vi "Creating_Backup_SQL.vi"(8 "error in":errorcluster, 10 "User level":i32, 11 "database in":T1) -> (0 "error out":errorcluster, 2 "User Level":i32, 3 "Database out":T1)   [LabVIEW 2017]
doc: "This vi we used to create SQL backup and delete that backup from SQL. This backup is moved to to CSV file.."
uses:
  <vilib>/addons/database/Connection.llb/Conn ObjectReference.ctl
  <vilib>/Utility/config.llb/Read Key (Path).vi
  <vilib>/Utility/config.llb/Read Key (Double).vi
  <vilib>/Utility/config.llb/Read Key (Boolean).vi
  <vilib>/Utility/file.llb/Write Delimited Spreadsheet (string).vi
  <vilib>/addons/database/NI_Database_API.lvlib
  <vilib>/Utility/config.llb/NI_LVConfig.lvlib
panel:
  out "Get Backup\nTreshold Time":timestamp caption="Get Backup Treshold Time"
  out "Backup Treshold Days":u32
  out "From Date":string
  in  "TO DATE":timestamp format="%<%d/%m/%Y>T"
  in  "FROM DATE":timestamp format="%<%d/%m/%Y>T"
  out "x*y":dbl
  out "x-y 3":dbl
  out "Backup Treshold Time":timestamp
  out "x-y":dbl
  out "Current Time":timestamp
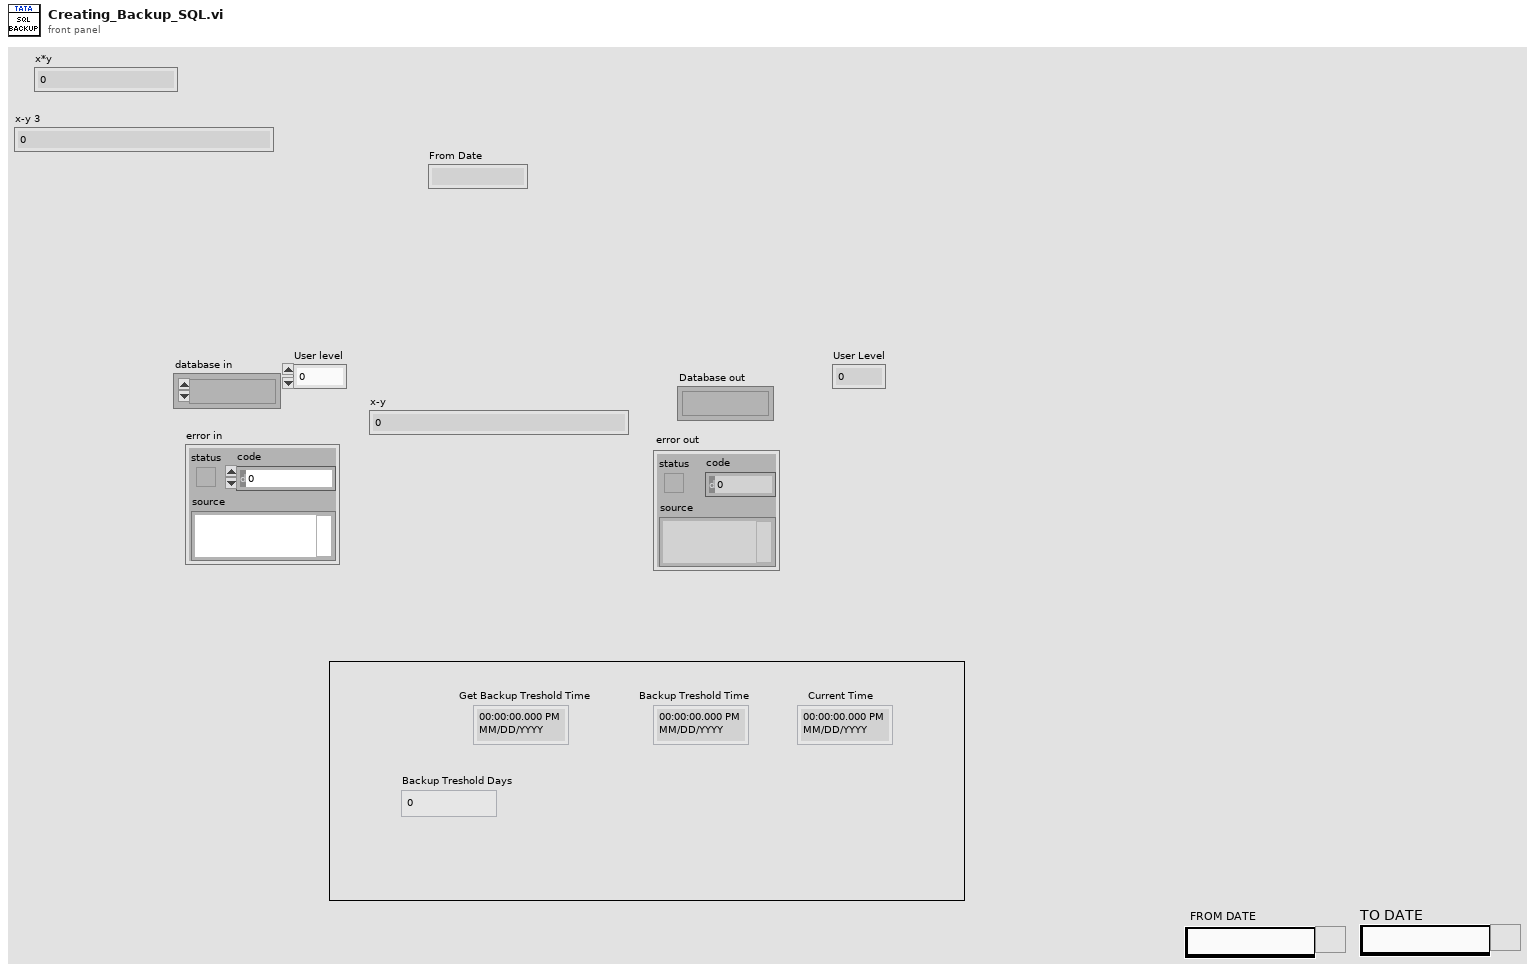
[diagram p1: front panel]
types:
  T1 = typedef "NI_Database_API.lvlib/Conn ObjectReference.ctl" = refnum<k1>
  T2 = enum32{"invalid app kind", "Development System", "Run Time System", "Student Edition", "Embedded LabVIEW", "Evaluation", "Custom"}
  T3 = typedef "NI_LVConfig.lvlib/Config Data RefNum.ctl" = refnum<k1>
  T4 = typedef "LVDateTimeRec.ctl" = cluster{"fractional second":dbl, "second":i32, "minute":i32, "hour":i32, "day of month":i32, "month":i32, "year":i32, "day of week":i32, "day of year":i32, "DST":i32}
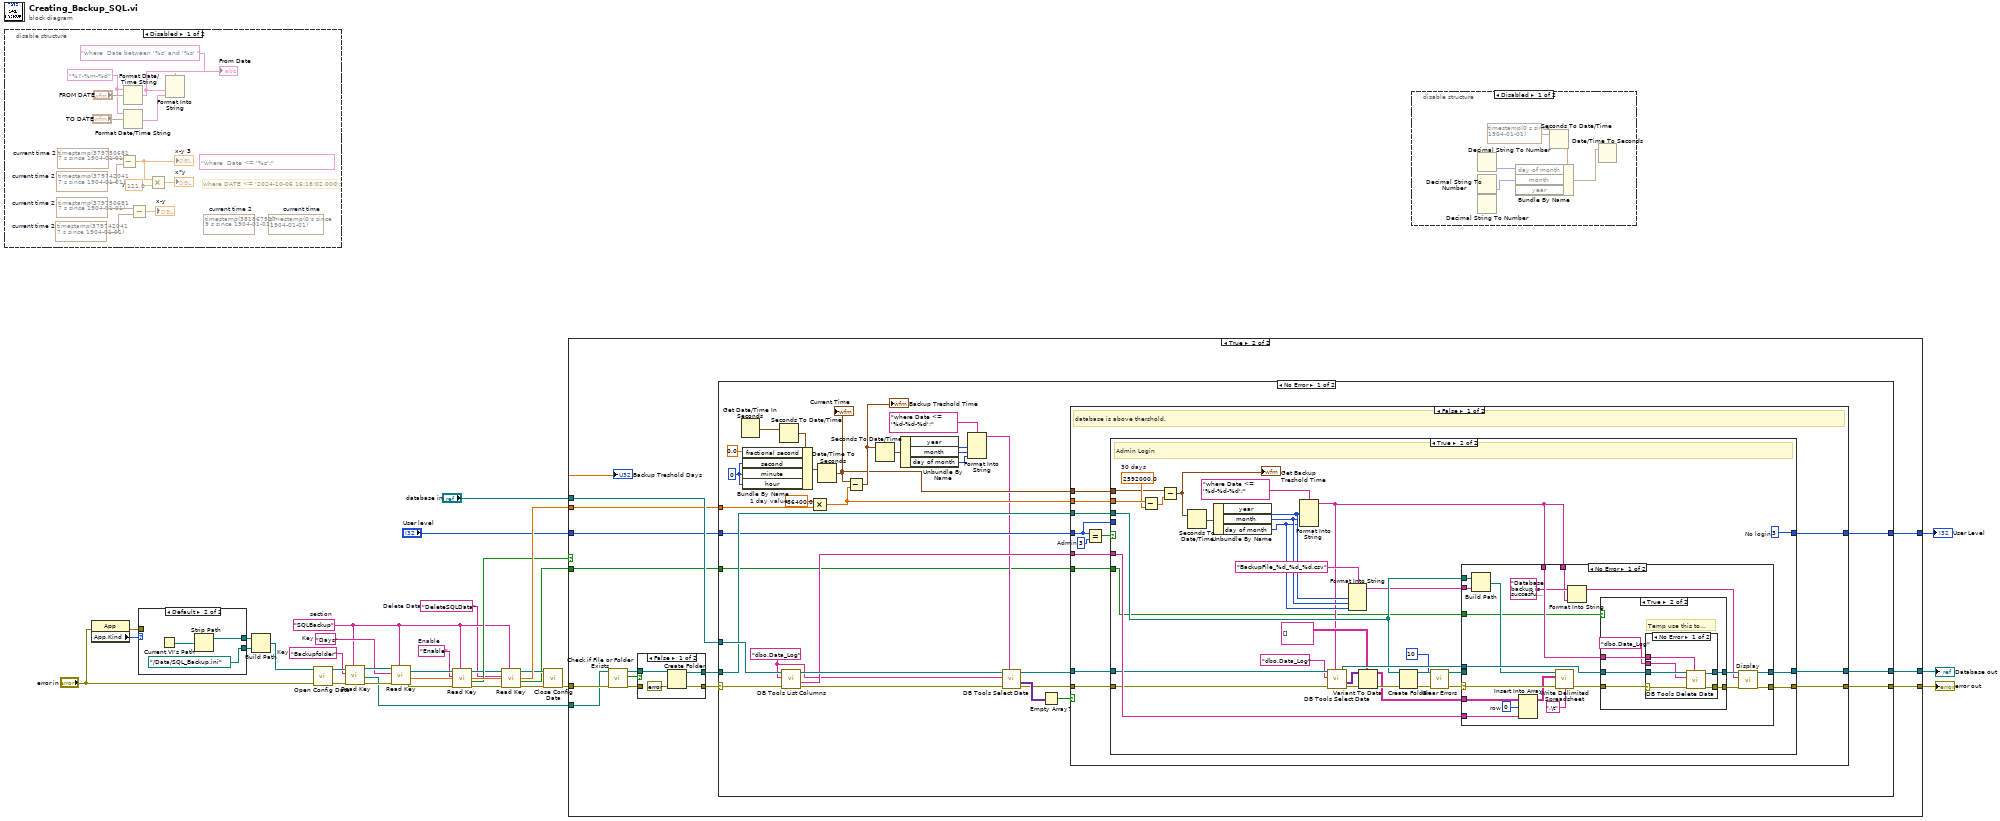
[diagram p0: block diagram]
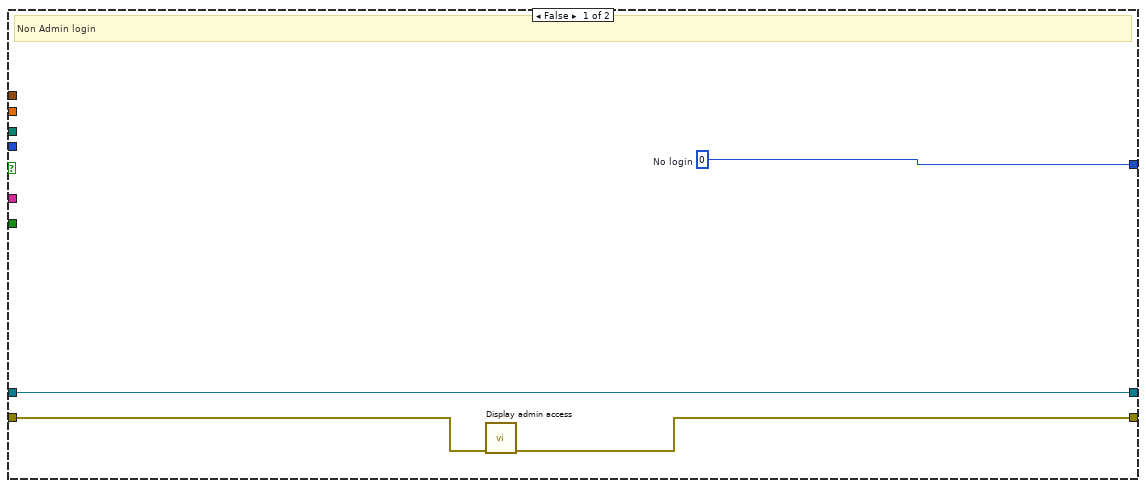
[diagram p4: hidden frame]
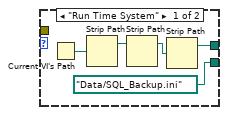
[diagram p12: hidden frame]
diagram:
  w2 = "DeleteSQLData"  # Delete Data
  w9 = "Enable"  # Enable
  w20 = "Days"  # Key
  w21 = "Backupfolder"  # Key
  w3 = "SQLBackup"  # section
  n1 = disable-structure shown="Disabled" {
    frame Disabled {
      w32 = "%Y-%m-%d"
      w39 = 121.0  # y
      w41 = timestamp(3797420417.197 s since 1904-01-01)  # current time 2
      w42 = timestamp(3797506817.197 s since 1904-01-01)  # current time 2
      (unwired) "where  Date <= '%s';" ("format string")
      (unwired) timestamp(3818675179.6780734 s since 1904-01-01)  # current time 2
      w44 = timestamp(3797420417.197 s since 1904-01-01)  # current time 2
      w45 = timestamp(3797506817.197 s since 1904-01-01)  # current time 2
      (unwired) timestamp(0 s since 1904-01-01)  # current time
      # "where DATE <= '2024-10-06 16:18:02.000';"
      n2 = Subtract(x=w42, y=w41) -> (x-y=w40:dbl)
      "x-y 3" <- w40
      n3 = Format Date/Time String(time format string (%c)=w32, seconds (now)="FROM DATE") -> (date/time string=w37:string)  [unwired: 1 in]
      "From Date" <- w37
      n4 = Format Date/Time String(time format string (%c)=w32, seconds (now)="TO DATE") -> (date/time string=w36:string)  [unwired: 1 in]
      n5 = Subtract(x=w45, y=w44) -> (x-y=→"x-y":dbl)
      n6 = Multiply(x=w40, y=w39) -> (x*y=→"x*y":dbl)
      n7 = Format Into String(format string="where  Date between '%s' and '%s' ", w37, w36) -> ()  [unwired: 2 in, 2 out]
    }
    frame Enabled {
    }
  }
  n8 = property class="App"(error in="error in") -> (error out=w28:errorcluster, "App.Kind"=w29:T2)  [unwired: 1 in, 1 out]
  n9 = case shown="Default" w29 {
    tunnel: [w47 w52] -> w27
    tunnel: w28 -> [_ _]
    tunnel: [path "Data/SQL_Backup.ini" ("path") path "../Data/SQL_Backup.ini" ("path")] -> w26
    frame "Run Time System" {
      n10 = Current VI's Path() -> (path=w50:path)
      n11 = Strip Path(path=w50) -> (stripped path=w49:path)  [unwired: 1 out]
      n12 = Strip Path(path=w49) -> (stripped path=w48:path)  [unwired: 1 out]
      n13 = Strip Path(path=w48) -> (stripped path=w47:path)  [unwired: 1 out]
    }
    frame Default {
      n14 = Current VI's Path() -> (path=w53:path)
      n15 = Strip Path(path=w53) -> (stripped path=w52:path)  [unwired: 1 out]
    }
  }
  n16 = Build Path(base path=w27, name or relative path=w26) -> (appended path=w17:path)
  n17 = call <vilib>:"Open Config Data.vi"("error in (no error)"="error in", "configuration file path"=w17) -> ("error out"=w25:errorcluster, "refnum"=w24:T3)  [unwired: 7 in, 1 out]
  n18 = call-poly <vilib>:"Read Key.vi"("section"=w3, "error in (no error)"=w25, "key"=w21, "refnum"=w24) -> ("error out"=w22:errorcluster, "value"=w16:path, "refnum out"=w23:T3)  [unwired: 4 in, 1 out]
  n19 = call-poly <vilib>:"Read Key.vi"("section"=w3, "error in (no error)"=w22, "key"=w20, "refnum"=w23) -> ("error out"=w11:errorcluster, "value"=w14:dbl, "refnum out"=w10:T3)  [unwired: 4 in, 1 out]
  n20 = call-poly <vilib>:"Read Key.vi"("section"=w3, "error in (no error)"=w11, "key"=w9, "refnum"=w10) -> ("error out"=w7:errorcluster, "value"=w8:bool, "refnum out"=w5:T3)  [unwired: 4 in, 1 out]
  n21 = call-poly <vilib>:"Read Key.vi"("section"=w3, "error in (no error)"=w7, "key"=w2, "refnum"=w5) -> ("error out"=w6:errorcluster, "value"=w1:bool, "refnum out"=w4:T3)  [unwired: 4 in, 1 out]
  n22 = call <vilib>:"Close Config Data.vi"("error in (no error)"=w6, "refnum"=w4) -> ("error out"=w18:errorcluster)  [unwired: 8 in, 1 out]
  n23 = case shown="True" w8 {
    tunnel: [w55 w65] -> w31
    tunnel: [w54 w64] -> w30
    tunnel: w18 -> [w55 w63]
    tunnel: w16 -> [_ w62]
    tunnel: "database in" -> [w54 w61]
    tunnel: w14 -> [_ w60]
    tunnel: "User level" -> [w56 w59]
    tunnel: [w56 w58] -> w12
    tunnel: w1 -> [_ w57]
    frame False {
      # "Bypass check"
    }
    frame True {
      n24 = call <vilib>:"Check if File or Folder Exists.vi"("error in (no error)"=w63, "path"=w62) -> ("error out"=w69:errorcluster, "file or folder exists?"=w70:bool, "dup path"=w68:path)  [unwired: 7 in]
      n25 = case shown="False" w70 {
        tunnel: w69 -> [_ w199]
        tunnel: w68 -> [w198 w200]
        tunnel: [w196 w200] -> w67
        tunnel: [w195 w199] -> w66
        frame False {
          n26 = Create Folder(path (use dialog)=w198, error in=errorcluster {"status"=FALSE, "code"=0, "source"=""}) -> (created path=w196:path, error out=w195:errorcluster)  [unwired: 1 in, 1 out]
        }
        frame True {
        }
      }
      n27 = case shown="No Error" w66 {
        selector: w66 -> [w100 w194]
        tunnel: w61 -> [w102 w193]
        tunnel: w67 -> [w97 _]
        tunnel: [w95 w194] -> w65
        tunnel: [w94 w193] -> w64
        tunnel: w60 -> [w86 _]
        tunnel: w59 -> [w83 w192]
        tunnel: [w75 w192] -> w58
        tunnel: w57 -> [w71 _]
        frame No Error {
          w87 = "dbo.Data_Log" ("table")
          w88 = 0 ("second")
          w93 = 86400.0  # 1 day value
          n28 = Get Date/Time In Seconds() -> (seconds since 1Jan1904=w90:timestamp)
          n29 = Seconds To Date/Time(time stamp (now)=w90) -> (date time rec=w91:T4)  [unwired: 1 in]
          n30 = Bundle By Name(cluster=w91, "fractional second"=0.0, "second"=w88, "minute"=w88, "hour"=w88) -> (w92:T4)
          n31 = call <vilib>:"DB Tools List Columns.vi"("error in (no error)"=w100, "table"=w87, "connection reference"=w102) -> ("error out"=w99:errorcluster, "columns"=w96:string[], "connection reference out"=w101:T1)  [unwired: 1 in, 1 out]
          n32 = Multiply(x=w93, y=w86) -> (x*y=w76:dbl)
          n33 = Date/Time To Seconds(2:w92) -> (0:w73:timestamp)  [unwired: 1 in]
          "Current Time" <- w73
          n34 = Subtract(x=w73, y=w76) -> (x-y=w74:timestamp)
          "Backup Treshold Time" <- w74
          n35 = Seconds To Date/Time(time stamp (now)=w74) -> (date time rec=w78:T4)  [unwired: 1 in]
          n36 = Unbundle By Name(w78) -> ("year"=w79:i32, "month"=w80:i32, "day of month"=w81:i32)
          n37 = Format Into String(format string="where Date <= '%d-%d-%d';", w79, w80, w81) -> (resulting string=w72:string)  [unwired: 2 in, 1 out]
          n38 = call <vilib>:"DB Tools Select Data.vi"("condition"=w72, "error in (no error)"=w99, "table"=w87, "connection reference"=w101) -> ("error out"=w82:errorcluster, "data"=w85:variant[][], "connection reference out"=w98:T1)  [unwired: 2 in]
          n39 = Empty Array?(array=w85) -> (empty?=w84:bool)
          n40 = case shown="False" w84 {
            tunnel: w98 -> [w115 w191]
            tunnel: w97 -> [w114 _]
            tunnel: w96 -> [w113 _]
            tunnel: [w112 w190] -> w95
            tunnel: [w111 w191] -> w94
            tunnel: w83 -> [w105 w189]
            tunnel: w82 -> [w110 w190]
            tunnel: w76 -> [w109 _]
            tunnel: w73 -> [w108 _]
            tunnel: [w104 w189] -> w75
            tunnel: w71 -> [w103 _]
            frame False {
              w107 = 3  # Admin
              # "database is above thershold."
              n41 = Equal?(x=w105, y=w107) -> (x = y?=w106:bool)
              n42 = case shown="True" w106 {
                tunnel: w115 -> [w119 w147]
                tunnel: w114 -> [_ w131]
                tunnel: w113 -> [_ w151]
                tunnel: [w118 w150] -> w112
                tunnel: [w119 w149] -> w111
                tunnel: w110 -> [w117 w143]
                tunnel: w109 -> [_ w142]
                tunnel: w108 -> [_ w139]
                tunnel: w105 -> [_ _]
                tunnel: [w116 w127] -> w104
                tunnel: w103 -> [_ w120]
                frame False {
                  w116 = 0  # No login
                  # "Non Admin login"
                  n43 = call "Display admin access"("error in (no error)"=w117) -> ("error out"=w118:errorcluster)  [unwired: 9 in, 1 out]
                }
                frame True {
                  w127 = 3  # No login
                  w141 = 2592000.0  # 30 days
                  # "Admin Login"
                  n44 = Subtract(x=w142, y=w141) -> (x-y=w140:dbl)
                  n45 = Subtract(x=w139, y=w140) -> (x-y=w122:timestamp)
                  "Get Backup\nTreshold Time" <- w122
                  n46 = Seconds To Date/Time(time stamp (now)=w122) -> (date time rec=w137:T4)  [unwired: 1 in]
                  n47 = Unbundle By Name(w137) -> ("year"=w134:i32, "month"=w133:i32, "day of month"=w132:i32)
                  n48 = Format Into String(format string="where Date <= '%d-%d-%d';", w134, w133, w132) -> (resulting string=w121:string)  [unwired: 2 in, 1 out]
                  n49 = call <vilib>:"DB Tools Select Data.vi"("condition"=w121, "error in (no error)"=w143, "table"="dbo.Data_Log", "connection reference"=w147) -> ("error out"=w144:errorcluster, "data"=w136:variant[][], "connection reference out"=w148:T1)  [unwired: 2 in]
                  n50 = Format Into String(format string="BackupFile_%d_%d_%d.csv", w134, w133, w132) -> (resulting string=w126:string)  [unwired: 2 in, 1 out]
                  n51 = Variant To Data(error in=w144, type=string[][] [], Variant=w136) -> (data=w128:string[][], error out=w130:errorcluster)
                  n52 = Create Folder(path (use dialog)=w131, error in=w130) -> (created path=w129:path, error out=w125:errorcluster)  [unwired: 1 in, 1 out]
                  n53 = call <vilib>:"Clear Errors.vi"("error in (no error)"=w125, "specific error code to clear (0: all)"=10) -> ("error out"=w124:errorcluster)  [unwired: 4 in, 1 out]
                  n54 = case shown="No Error" w124 {
                    selector: w124 -> [w166 w188]
                    tunnel: w148 -> [w167 w187]
                    tunnel: w151 -> [w161 _]
                    tunnel: [w163 w188] -> w150
                    tunnel: [w168 w187] -> w149
                    tunnel: w129 -> [_ _]
                    tunnel: w128 -> [w160 _]
                    tunnel: w121 -> [w165 _]
                    tunnel: w131 -> [w158 _]
                    tunnel: w126 -> [w157 _]
                    tunnel: w121 -> [w154 _]
                    tunnel: w120 -> [w152 _]
                    frame No Error {
                      w162 = 0  # row
                      n55 = Build Path(base path=w158, name or relative path=w157) -> (appended path=w156:path)
                      n56 = Insert Into Array(array=w160, index (row)=w162, new element=w161) -> (w159:string[][])  [unwired: 1 in]
                      n57 = call-poly <vilib>:"Write Delimited Spreadsheet.vi"("file path (dialog if empty)"=w156, "2D data"=w159, "error in (no error)"=w166, "delimiter (\\t)"=",\t" ("delimiter (\\t)")) -> ("error out"=w169:errorcluster)  [unwired: 10 in, 1 out]
                      n58 = Format Into String(format string="Database backup is succesfully taken. for date before = %s", w154) -> (resulting string=w153:string)  [unwired: 2 in, 1 out]
                      n59 = case shown="True" w152 {
                        tunnel: w169 -> [w172 w178]
                        tunnel: [w171 w177] -> w168
                        tunnel: w167 -> [w171 w176]
                        tunnel: w165 -> [_ w175]
                        tunnel: [w172 w174] -> w164
                        frame False {
                        }
                        frame True {
                          # "Temp use this to\ncheck backup before\nimplimenting."
                          n60 = case shown="No Error" w178 {
                            selector: w178 -> [w184 w186]
                            tunnel: [w183 w186] -> w174
                            tunnel: [w182 w185] -> w177
                            tunnel: w176 -> [w181 w185]
                            tunnel: w175 -> [w180 _]
                            tunnel: "dbo.Data_Log" ("table") -> [w179 _]
                            frame No Error {
                              n61 = call <vilib>:"DB Tools Delete Data.vi"("condition"=w180, "error in (no error)"=w184, "table"=w179, "connection reference"=w181) -> ("error out"=w183:errorcluster, "connection reference out"=w182:T1)  [unwired: 6 in]
                            }
                            frame Error {
                            }
                          }
                        }
                      }
                      n62 = call "Display"("error in (no error)"=w164, "Message"=w153) -> ("error out"=w163:errorcluster)  [unwired: 8 in, 1 out]
                    }
                    frame Error {
                    }
                  }
                }
              }
            }
            frame True {
              # "\"Date_st2\" is not given column of data"
            }
          }
        }
        frame Error {
        }
      }
      "Backup Treshold Days" <- w60
    }
  }
  "Database out" <- w30
  "error out" <- w31
  "User Level" <- w12
  n63 = disable-structure shown="Disabled" {
    frame Disabled {
      n64 = Decimal String To Number() -> (number=w203:i32)  [unwired: 3 in, 1 out]
      n65 = Decimal String To Number() -> (number=w202:i32)  [unwired: 3 in, 1 out]
      n66 = Decimal String To Number() -> ()  [unwired: 3 in, 2 out]
      n67 = Seconds To Date/Time(time stamp (now)=timestamp(0 s since 1904-01-01)) -> (date time rec=w205:T4)  [unwired: 1 in]
      n68 = Bundle By Name(cluster=w205, "day of month"=w203, "month"=w202) -> (w204:T4)  [unwired: 1 in]
      n69 = Date/Time To Seconds(2:w204) -> ()  [unwired: 1 in, 1 out]
    }
    frame Enabled {
    }
  }
